vi "Save to TDMS.vi"(8 "error in (no error)":errorcluster, 11 "Logging Cluster":T1 {"Exp params"."TSFrames" min=1 step=1; "Exp params"."TSfps" min=0.001 max=90.0 step=0.001 format="%_4g"}) -> (0 "error out":errorcluster)   [LabVIEW 2020]
uses:
  _controls/Logging Cluster.ctl
  _controls/Exp Params.ctl
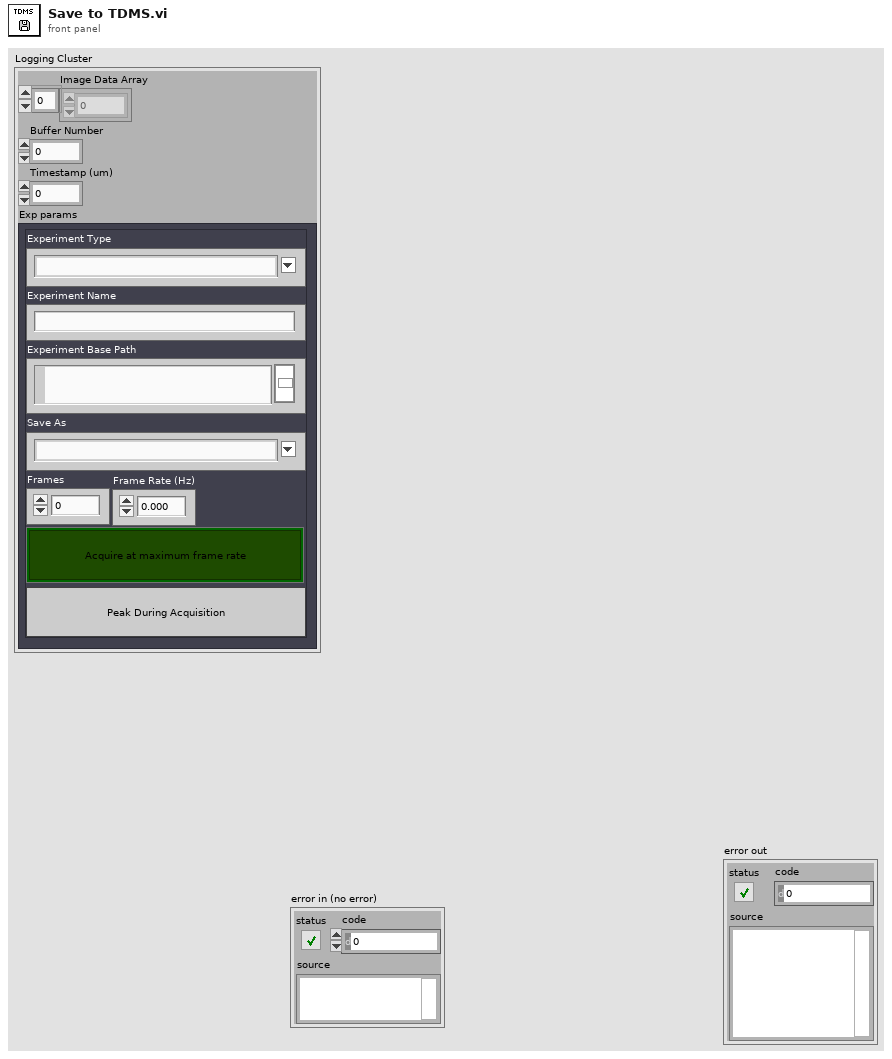
[diagram p1: front panel]
types:
  T1 = typedef "Logging Cluster.ctl" = cluster{"Image Data Array":u8[], "Buffer Number":i32, "Timestamp (um)":u64, "Exp params":T2}
  T2 = typedef "Exp Params.ctl" = cluster{"Experiment Type":string, "Experiment Name":string, "ExpPath":path, "Save As":string, "TSFrames":i32, "TSfps":dbl, "Streaming":bool, "tdms ref":refnum<k34>, "frame #":i64, "Full Path":path, "PeakOnQueue":bool}
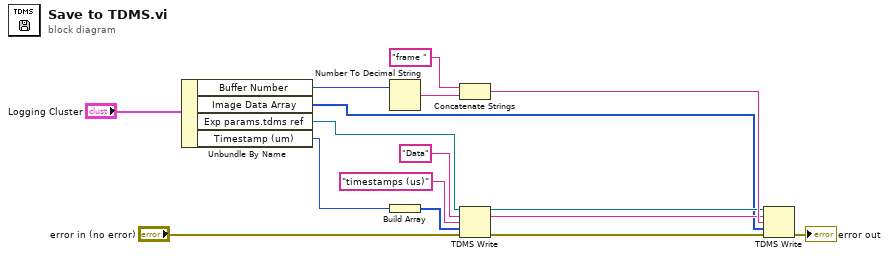
[diagram p0: block diagram]
diagram:
  n1 = Unbundle By Name("Logging Cluster") -> ("Buffer Number"=w7:i32, "Image Data Array"=w4:u8[], "Exp params.tdms ref"=w6:refnum<k34>, "Timestamp (um)"=w5:u64)
  n2 = Number To Decimal String(number=w7) -> (decimal integer string=w13:string)  [unwired: 1 in]
  n3 = Build Array(w5) -> (w1:u64[])
  n4 = Concatenate Strings("frame ", w13) -> (w12:string)
  n5 = TDMS Write(0:w6, 5:"Data" ("group name in (Untitled)"), 7:"timestamps (us)" ("group name in (Untitled)"), 9:w1, 11:"error in (no error)") -> (4:w11:refnum<k34>, 6:w10:string, 15:w9:errorcluster)  [unwired: 1 in, 1 out]
  n6 = TDMS Write(0:w11, 5:w10, 7:w12, 9:w4, 11:w9) -> (15:→"error out":errorcluster)  [unwired: 1 in, 3 out]
